vi "Tx-Mapping Detail's.vi"(7 "Data Cluster In":T1, 8 "error in (no error)":errorcluster) -> (0 "error out":errorcluster, 5 "Data Cluster Out":T1)   [LabVIEW 2021, in "Test Panel.lvlib"]
doc: "<b>Note:</b> This VI was modified by the <b>Validate DQMH Module</b> tool to turn off automatic error handling."
uses:
  Test Panel.lvlib
  Module Data--cluster.ctl
  GUI Ctrl Data's--Cluster.ctl
  Rx-Mapping Data.ctl
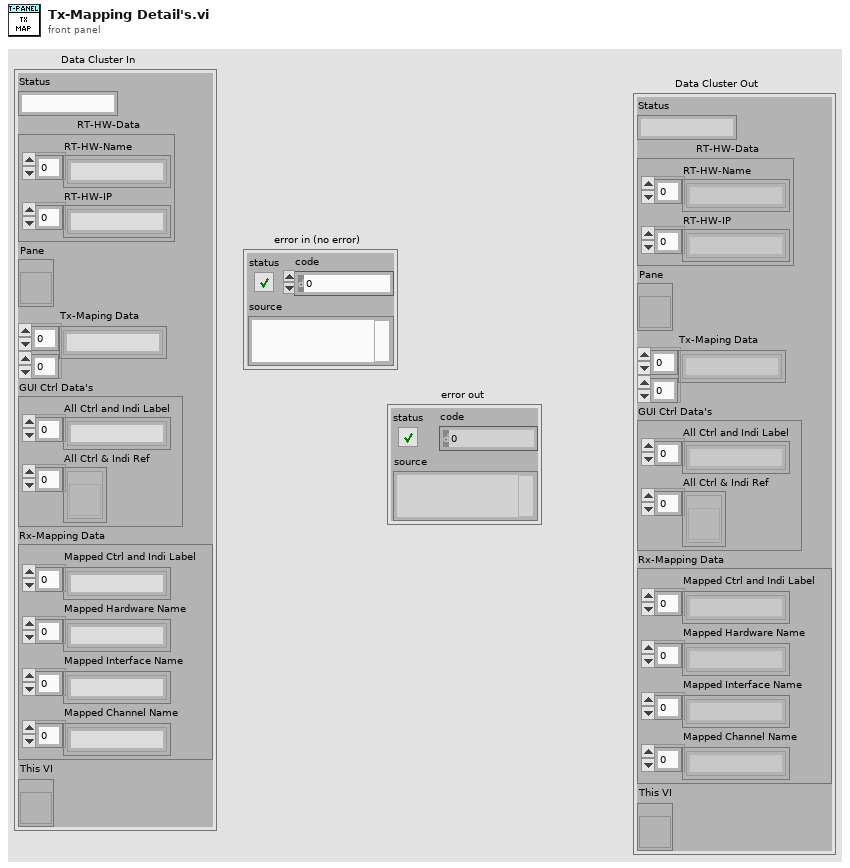
[diagram p1: front panel]
types:
  T1 = typedef "Test Panel.lvlib/Module Data--cluster.ctl" = cluster{"Status":string, "RT-HW-Data":cluster{"RT-HW-Name":string[], "RT-HW-IP":string[]}, "Pane":refnum<vi>, "Tx-Maping Data":string[][], "GUI Ctrl Data's":T2, "Rx-Mapping Data":T3, "This VI":refnum<vi>}
  T2 = typedef "Test Panel.lvlib/GUI Ctrl Data's--Cluster.ctl" = cluster{"All Ctrl and Indi Label":string[], "All Ctrl & Indi Ref":refnum<vi>[]}
  T3 = typedef "Test Panel.lvlib/Rx-Mapping Data.ctl" = cluster{"Mapped Ctrl and Indi Label":string[], "Mapped Hardware Name":string[], "Mapped Interface Name":string[], "Mapped Channel Name":string[]}
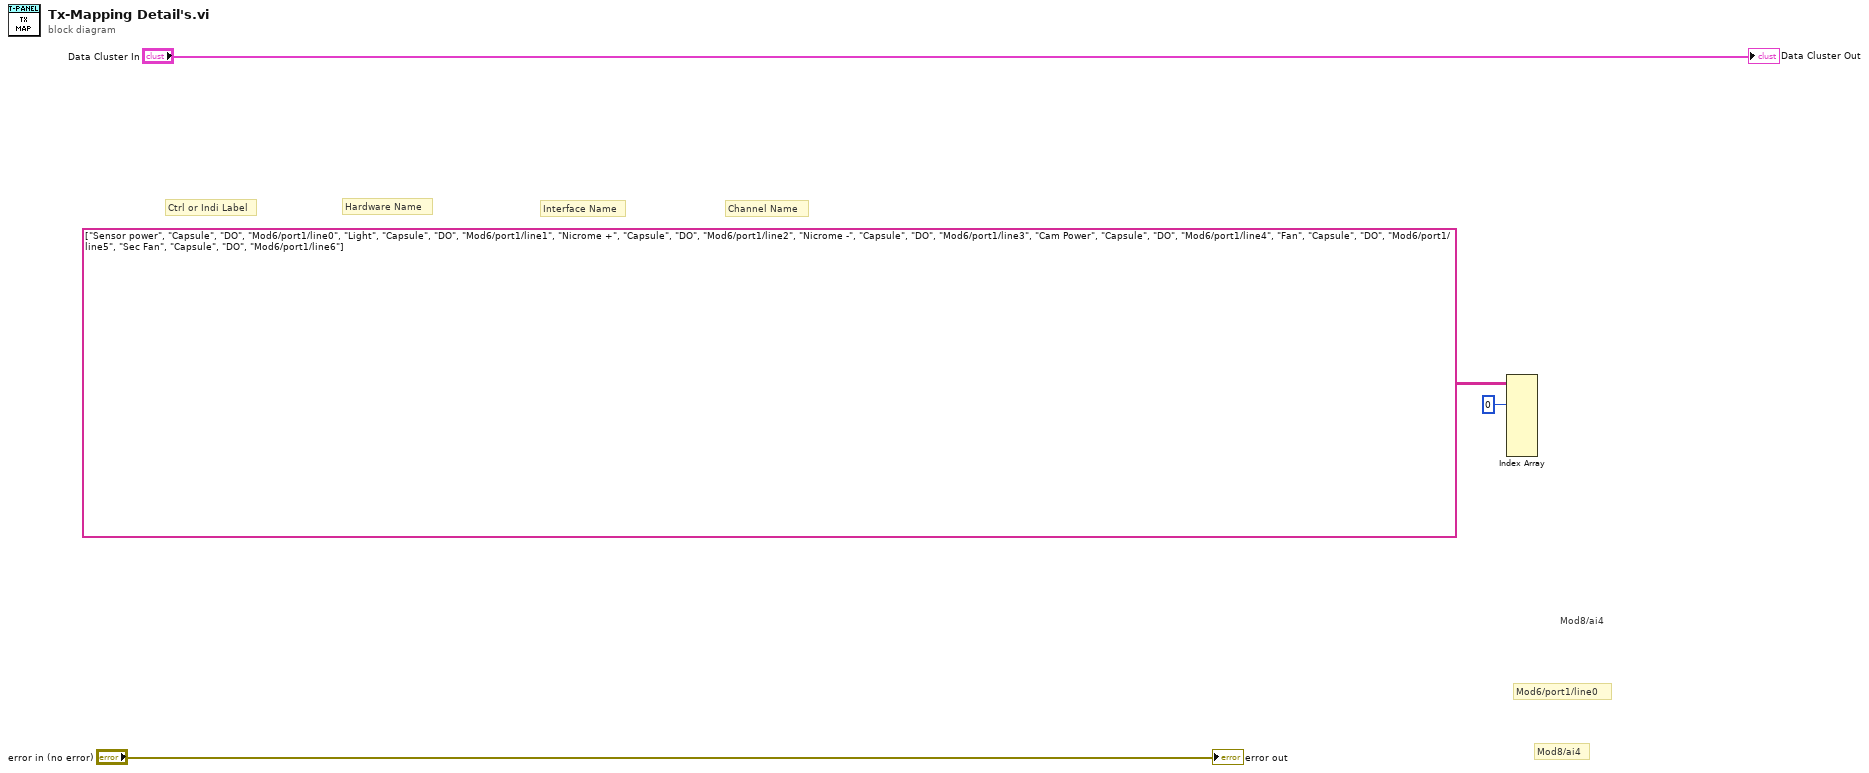
[diagram p0: block diagram]
diagram:
  # "Mod6/port1/line0"
  # "Mod8/ai4"
  # "Mod8/ai4"
  # "Channel Name"
  # "Ctrl or Indi Label"
  # "Interface Name"
  # "Hardware Name"
  n1 = Index Array(array=string[][] [["Sensor power", "Capsule", "DO", "Mod6/port1/line0"], ["Light", "Capsule", "DO", "Mod6/port1/line1"], ["Nicrome +", "Capsule", "DO", "Mod6/port1/line2"], ["Nicrome -", "Capsule", "DO", "Mod6/port1/line3"], ["Cam Power", "Capsule", "DO", "Mod6/port1/line4"], ["Fan", "Capsule", "DO", "Mod6/port1/line5"], ["Sec Fan", "Capsule", "DO", "Mod6/port1/line6"]], index (col) #1=0 ("index (col)")) -> ()  [unwired: 7 in, 4 out]
  "Data Cluster Out" <- "Data Cluster In"
  "error out" <- "error in (no error)"
